vi "navX Read Values.vi"() -> (0 "Connected":bool)   [LabVIEW 2016]
uses:
  Robot Global Data.vi
  <vilib>/Rock Robotics/Network Tables/NT Write Number.vi
panel:
  out "Self Test Status":T1
  out "Sensor Status":T2
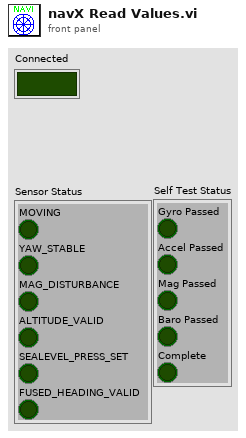
[diagram p1: front panel]
types:
  T1 = cluster{"Gyro Passed":bool, "Accel Passed":bool, "Mag Passed":bool, "Baro Passed":bool, "Complete":bool}
  T2 = cluster{"MOVING":bool, "YAW_STABLE":bool, "MAG_DISTURBANCE":bool, "ALTITUDE_VALID":bool, "SEALEVEL_PRESS_SET":bool, "FUSED_HEADING_VALID":bool}
  T3 = typedef "FRIC_navX_DeviceNumbersTypeDef.ctl" = enum16{"Dev0", "Dev1", "Dev2", "Dev3"}
  T4 = typedef "Z900_navX_Flags_OpStatusTypeDef.ctl" = u8
  T5 = typedef "Z900_navX_Flags_CalibrationStatusTypeDef.ctl" = u8
  T6 = cluster{"Update Rate Hz":u8, "Accelerometer Full-Scale Range":u8, "Gyro Full-Scale Range":u16, "OP Status":T4, "Calibration Status":T5, "Sensor Status":cluster{"MOVING":bool, "YAW_STABLE":bool, "MAG_DISTURBANCE":bool, "ALTITUDE_VALID":bool, "SEALEVEL_PRESS_SET":bool, "FUSED_HEADING_VALID":bool}, "Self Test Status":cluster{"Gyro Passed":bool, "Accel Passed":bool, "Mag Passed":bool, "Baro Passed":bool, "Complete":bool}}
  T7 = cluster{"LinearAcceleration X":dbl, "LinearAcceleration Y":dbl, "LinearAcceleration Z":dbl}
  T8 = cluster{"Yaw":dbl, "Roll":dbl, "Pitch":dbl, "Heading":dbl, "Fused Heading":dbl}
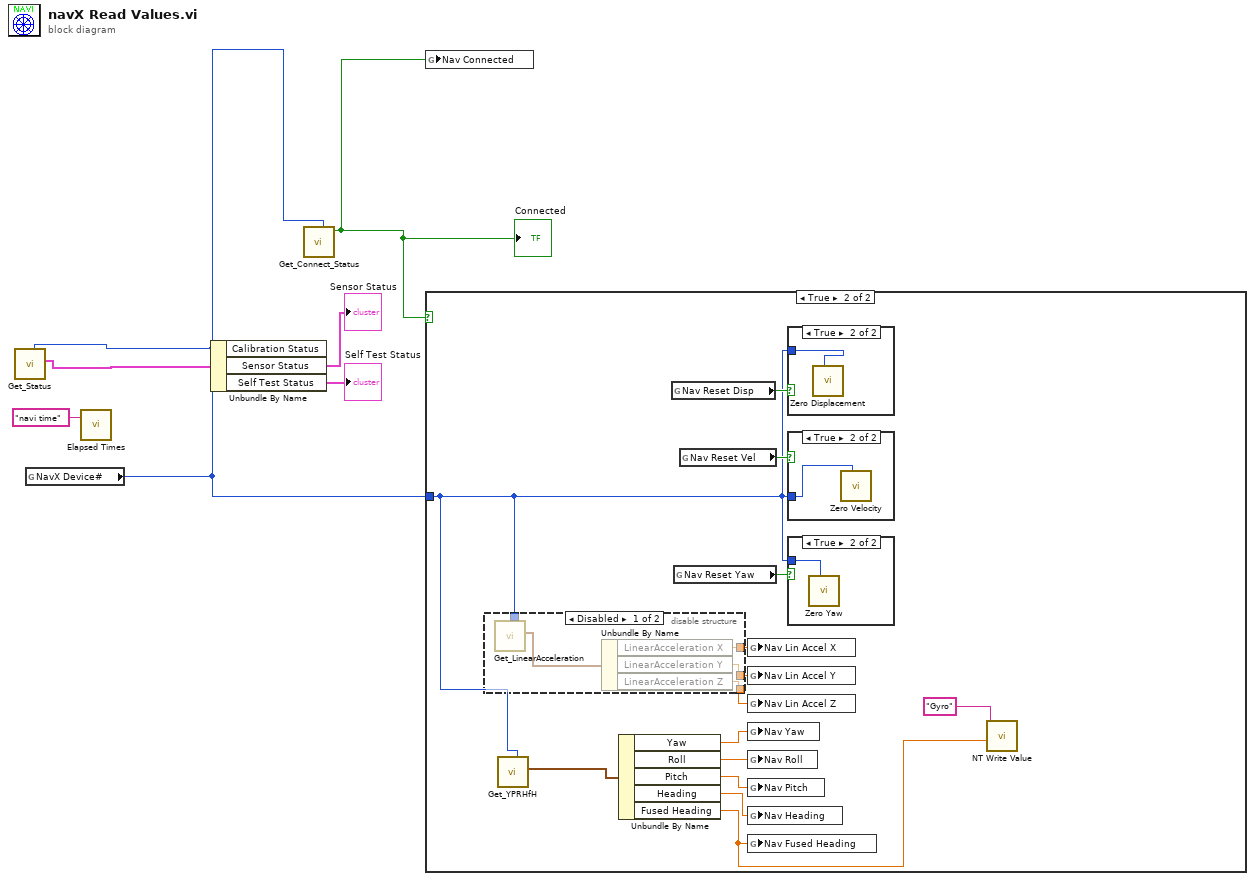
[diagram p0: block diagram]
diagram:
  n1 = global read "Robot Global Data.vi" "NavX Device#"() -> (w1:T3)
  n2 = call <vilib>:"Get_Status.vi"("Device Number"=w1) -> ("Status"=w3:T6)  [unwired: 10 in]
  n3 = call "Elapsed Times.vi"("Call Name"="navi time") -> ()  [unwired: 2 in, 1 out]
  n4 = Unbundle By Name(w3) -> ("Sensor Status"=→"Sensor Status":T2, "Self Test Status"=→"Self Test Status":T1)  [unwired: 1 out]
  n5 = call <vilib>:"Get_Connect_Status.vi"("Device Number"=w1) -> ("Connected"=w2:bool)  [unwired: 10 in]
  "Connected" <- w2
  n6 = global write "Robot Global Data.vi" "Nav Connected"(w2) -> ()
  n7 = case shown="True" w2 {
    tunnel: w1 -> [_ w11]
    frame False {
    }
    frame True {
      n8 = disable-structure shown="Disabled" {
        disable-tunnel: [w25 _] -> w14
        disable-tunnel: [w24 _] -> w13
        disable-tunnel: [w23 _] -> w12
        disable-tunnel: w11 -> [w21 _]
        frame Disabled {
          n9 = call <vilib>:"Get_LinearAcceleration.vi"("Device Number"=w21) -> ("Linear Acceleration"=w22:T7)  [unwired: 10 in]
          n10 = Unbundle By Name(w22) -> ("LinearAcceleration X"=w25:dbl, "LinearAcceleration Y"=w23:dbl, "LinearAcceleration Z"=w24:dbl)
        }
        frame Enabled {
        }
      }
      n11 = call <vilib>:"Get_YPRHfH.vi"("Device Number"=w11) -> ("YRPHfH"=w10:T8)  [unwired: 10 in]
      n12 = Unbundle By Name(w10) -> ("Yaw"=w9:dbl, "Roll"=w17:dbl, "Pitch"=w16:dbl, "Heading"=w15:dbl, "Fused Heading"=w7:dbl)
      n13 = global read "Robot Global Data.vi" "Nav Reset Disp"() -> (w18:bool)
      n14 = global read "Robot Global Data.vi" "Nav Reset Yaw"() -> (w20:bool)
      n15 = global read "Robot Global Data.vi" "Nav Reset Vel"() -> (w19:bool)
      n16 = global write "Robot Global Data.vi" "Nav Lin Accel X"(w14) -> ()
      n17 = global write "Robot Global Data.vi" "Nav Lin Accel Y"(w12) -> ()
      n18 = global write "Robot Global Data.vi" "Nav Lin Accel Z"(w13) -> ()
      n19 = global write "Robot Global Data.vi" "Nav Yaw"(w9) -> ()
      n20 = global write "Robot Global Data.vi" "Nav Roll"(w17) -> ()
      n21 = global write "Robot Global Data.vi" "Nav Pitch"(w16) -> ()
      n22 = global write "Robot Global Data.vi" "Nav Heading"(w15) -> ()
      n23 = global write "Robot Global Data.vi" "Nav Fused Heading"(w7) -> ()
      n24 = case shown="True" w18 {
        tunnel: w11 -> [_ w26]
        frame False {
        }
        frame True {
          n25 = call <vilib>:"Zero Displacement.vi"("Device Number"=w26) -> ()  [unwired: 11 in]
        }
      }
      n26 = case shown="True" w19 {
        tunnel: w11 -> [_ w27]
        frame False {
        }
        frame True {
          n27 = call <vilib>:"Zero Velocity.vi"("Device Number"=w27) -> ()  [unwired: 11 in]
        }
      }
      n28 = case shown="True" w20 {
        tunnel: w11 -> [_ w28]
        frame False {
        }
        frame True {
          n29 = call <vilib>:"Zero Yaw.vi"("Device Number"=w28) -> ()  [unwired: 11 in]
        }
      }
      n30 = call-poly <vilib>:"NT Write Value.vi"("Numeric"=w7, "Name"="Gyro") -> ()  [unwired: 9 in, 1 out]
    }
  }
